vi "Variant Constant (null).vi"() -> (1 "null":variant)   [LabVIEW 2015]
doc: "Empty variant (void variant wrapped by variant) represents null on serialization."
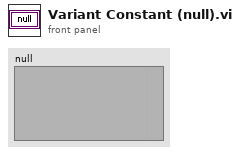
[diagram p1: front panel]
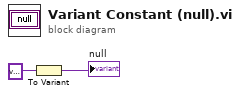
[diagram p0: block diagram]
diagram:
  n1 = To Variant(anything=variant) -> (Variant=→"null":variant)
